vi "SPU_Get_Sampling_Rawdata.vi"(7 "错误输入（无错误）":errorcluster, 10 "SPU":refnum<k24>) -> (0 "error out":errorcluster caption="error IO", 1 "monitor":sgl[](array[numeric]), 2 "trigger":sgl[](array[numeric]), 3 "SPU out":refnum<k24>)   [LabVIEW 2017]
uses:
  D:/test/PDLSTS/LV_PDL LvVer17.0/LV_PDL_x64/DLL/InstrumentDLL.dll
  DLL/InstrumentDLL.dll
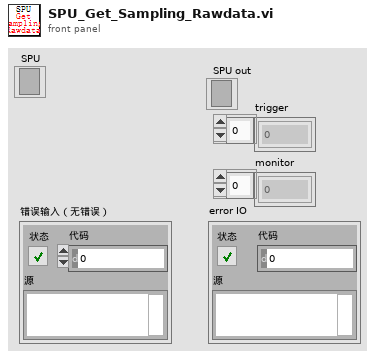
[diagram p1: front panel]
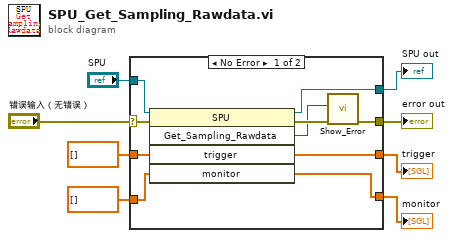
[diagram p0: block diagram]
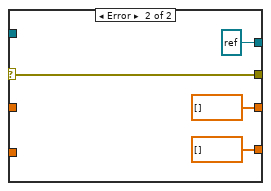
[diagram p2: hidden frame]
diagram:
  n1 = case shown="No Error" "错误输入（无错误）" {
    selector: "错误输入（无错误）" -> [w14 w22]
    tunnel: [w16 w22] -> w6
    tunnel: [w15 refnum<k24> refnum ("new reference")] -> w7
    tunnel: "SPU" -> [w13 _]
    tunnel: [w12 sgl[] [] ("trigger")] -> w4
    tunnel: [w11 sgl[] [] ("monitor")] -> w3
    tunnel: sgl[] [] ("monitor") -> [w10 _]
    tunnel: sgl[] [] ("trigger") -> [w9 _]
    frame No Error {
      n2 = invoke class="SPU" method="Get_Sampling_Rawdata"(reference=w13, error in=w14, "trigger"=w9, "monitor"=w10) -> (reference out=w15:refnum<k24>, error out=w18:errorcluster, "Get_Sampling_Rawdata"=w17:i32, "trigger"=w12:sgl[], "monitor"=w11:sgl[])  [unwired: 1 in]
      n3 = call "Show_Error.vi"("error in (no error)"=w18, "Error"=w17) -> ("error out"=w16:errorcluster)  [unwired: 9 in]
    }
    frame Error {
    }
  }
  "SPU out" <- w7
  "error out" <- w6
  "trigger" <- w4
  "monitor" <- w3
